vi "Temperature Converter Internals.vi"(1 "Boolean":bool, 2 "Temperaturee (C)":dbl) -> (0 "Numeric":dbl)   [LabVIEW 2023]
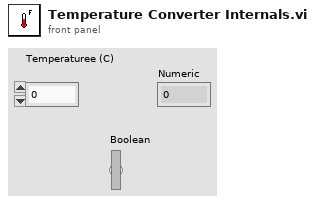
[diagram p1: front panel]
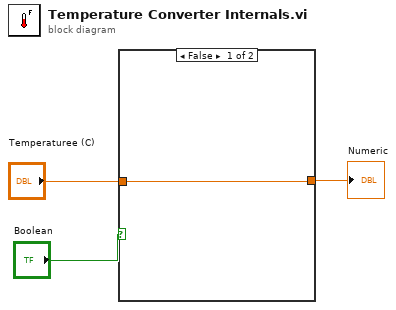
[diagram p0: block diagram]
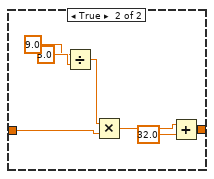
[diagram p2: hidden frame]
diagram:
  n1 = case shown="False" "Boolean" {
    tunnel: [w4 w11] -> w1
    tunnel: "Temperaturee (C)" -> [w4 w9]
    frame False {
    }
    frame True {
      n2 = Divide(x=9.0, y=5.0) -> (x/y=w8:dbl)
      n3 = Multiply(x=w8, y=w9) -> (x*y=w10:dbl)
      n4 = Add(x=w10, y=32.0) -> (x+y=w11:dbl)
    }
  }
  "Numeric" <- w1
